vi "Select Exception Objects.vi"(10 "Response":refnum<class "Response.lvclass">, 11 "Processing":refnum<class "Processing.lvclass">) -> (3 "Updated Inputs":refnum<class "Processing.lvclass">, 7 "Trace Message":string)   [LabVIEW 2020, in "HTTP Server.lvlib" / "Server.lvclass"]
uses:
  Server.lvclass
  Processing/Processing.lvclass
  Processing/Processing.lvclass/Processing.ctl
  Server.lvclass/Server.ctl
  <vilib>/IlluminatedG/IG HTTP Utils/HTTP Utils/Response/Response.lvclass
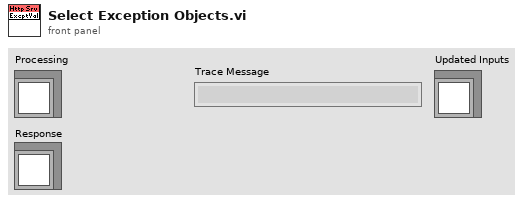
[diagram p1: front panel]
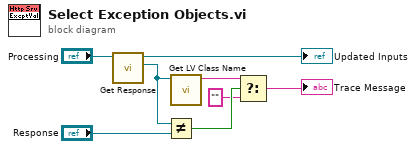
[diagram p0: block diagram]
diagram:
  n1 = call "Get Response.vi"("Processing in"="Processing") -> ("Response"=w3:refnum<class "Response.lvclass">, "Processing out"=→"Updated Inputs":refnum<class "Processing.lvclass">)  [unwired: 9 in]
  n2 = Not Equal?(x=w3, y="Response") -> (x != y?=w7:bool)
  n3 = call <vilib>:"Get LV Class Name.vi"("object"=w3) -> ("class name"=w8:string)  [unwired: 9 in, 1 out]
  n4 = Select(t=w8, s=w7, f="") -> (s? t:f=→"Trace Message":string)
